vi "GetQ_array string.vi"(8 "error in (no error)":errorcluster, 10 "QNames":string[](array[string])) -> (0 "error out":errorcluster, 1 "foundArray":bool[](array[boolean]), 2 "QueueArray":refnum<queue>[](array[refnum]))   [LabVIEW 2020, in "QDict.lvlib"]
doc: "Developed by Kevin Thompson\nkevin@thompsonengineering.net\n\nCopyright 2021\nThompson Engineering, LLC"
uses:
  QDict.lvlib
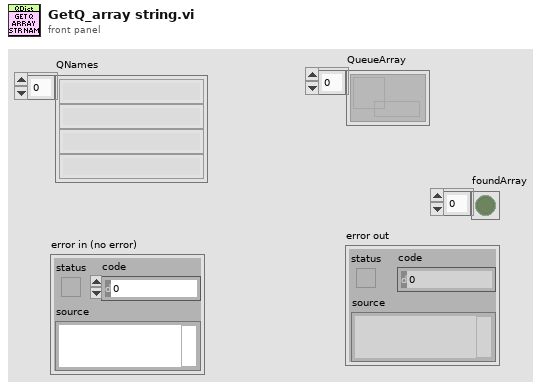
[diagram p1: front panel]
types:
  T1 = typedef "TD Dynamic CVT DVR--ref.ctl" = refnum<data-value>
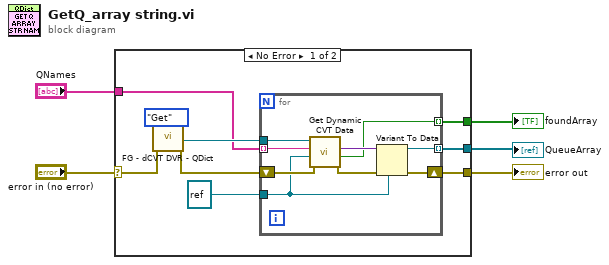
[diagram p0: block diagram]
diagram:
  n1 = case shown="No Error" "error in (no error)" {
    selector: "error in (no error)" -> [w13 w24]
    tunnel: "QNames" -> [w10 _]
    tunnel: [w9 _] -> w3
    tunnel: [w7 _] -> w2
    tunnel: [w6 w24] -> w1
    frame No Error {
      n2 = call "FG - dCVT DVR - QDict.vi"("error in (no error)"=w13, "Action (Get)"=enum16{"Init", "Get", "Set"}."Get") -> ("dCVT QMH out"=w12:T1, "error out"=w11:errorcluster)  [unwired: 7 in]
      n3 = for {
        tunnel: w12 -> [w23]
        tunnel: w10 -> [w19] mode=indexing
        tunnel: [w18] -> w9 mode=indexing
        tunnel: [w16] -> w7 mode=indexing
        shift-right: [w17] -> w6
        shift-left: w11 -> [w22]
        tunnel: refnum<queue> refnum ("queue out") -> [w15]
        n4 = call <vilib>:"Get Dynamic CVT Data.vi"("error in (no error)"=w22, "default value (empty variant)"=w15, "DataName"=w19, "dCVT DVR"=w23) -> ("error out"=w21:errorcluster, "found"=w16:bool, "value"=w20:variant)  [unwired: 4 in, 1 out]
        n5 = Variant To Data(error in=w21, type=w15, Variant=w20) -> (data=w18:refnum<queue>, error out=w17:errorcluster)
      }
    }
    frame Error {
    }
  }
  "error out" <- w1
  "QueueArray" <- w3
  "foundArray" <- w2
